vi "Get Abundant Numbers.vi"(11 "Limit":i32) -> (3 "Abundant Numbers":i32[](array[numeric]))   [LabVIEW 2013, in "Problem 23.lvlib"]
uses:
  Problem 23.lvlib
  Problem 21/Problem 21.lvlib
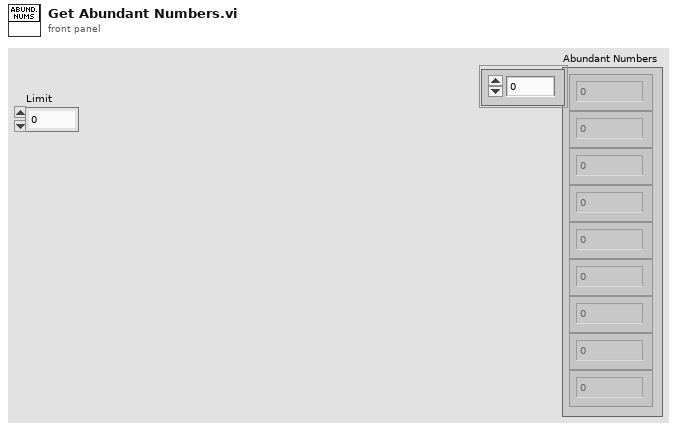
[diagram p1: front panel]
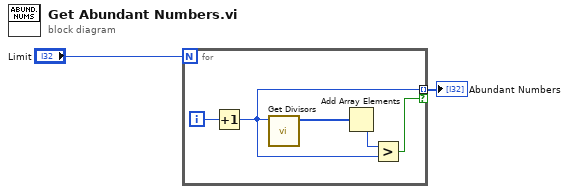
[diagram p0: block diagram]
diagram:
  n1 = for {
    N: "Limit" -> [_]
    tunnel: [w4] -> w1 mode=indexing if=w3
    i -> [w7]
    n2 = Increment(x=w7) -> (x+1=w4:i32)
    n3 = call "Get Divisors.vi"("Number"=w4) -> ("Divisors"=w6:i32[])  [unwired: 10 in]
    n4 = Add Array Elements(numeric array=w6) -> (sum=w5:i32)
    n5 = Greater?(x=w5, y=w4) -> (0:w3:bool)
  }
  "Abundant Numbers" <- w1
